vi "Write DeviceID.vi"(10 "DeviceID":T1, 11 "Device DDS Communications in":refnum<class "Device DDS Communications.lvclass">) -> (3 "Device DDS Communications out":refnum<class "Device DDS Communications.lvclass">)   [LabVIEW 2018, in "Device DDS Communications Framework.lvlib" / "Device DDS Communications.lvclass"]
uses:
  Device DDS Communications.lvclass
  <vilib>/ORNL/CSEISMIC DDS/CSEISMIC DDS Base/Data Types/Controls/DeviceID.ctl
  Device DDS Communications.lvclass/Device DDS Communications.ctl
  <vilib>/ORNL/CSEISMIC DDS/CSEISMIC DDS Base/CSEISMIC DDS.lvclass
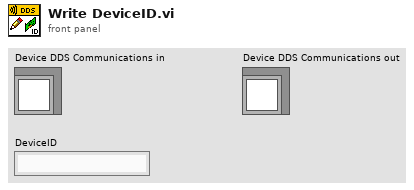
[diagram p1: front panel]
types:
  T1 = typedef "CSEISMIC DDS.lvlib/CSEISMIC DDS.lvclass/DeviceID.ctl" = string
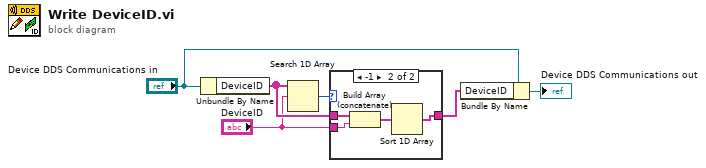
[diagram p0: block diagram]
diagram:
  n1 = Unbundle By Name("Device DDS Communications in") -> ("DeviceID"=w5:T1[])
  n2 = Search 1D Array(1D array=w5, element="DeviceID") -> (index of element=w4:i32)  [unwired: 1 in]
  n3 = case shown="-1" w4 {
    tunnel: w5 -> [w7 w11]
    tunnel: "DeviceID" -> [_ w10]
    tunnel: [w7 w8] -> w1
    frame 0, Default {
    }
    frame -1 {
      n4 = Build Array (concatenate)(w11, w10) -> (w9:T1[])
      n5 = Sort 1D Array(array=w9) -> (sorted array=w8:T1[])
    }
  }
  n6 = Bundle By Name(cluster="Device DDS Communications in", "DeviceID"=w1) -> (→"Device DDS Communications out":refnum<class "Device DDS Communications.lvclass">)
